vi "Build.vi"() -> ()   [LabVIEW 2014]
uses:
  <vilib>/AppBuilder/AB_API_Simple/Build Specification Version.ctl
  <vilib>/AppBuilder/AB_API_Simple/NI_App_Builder_API.lvlib
  <vilib>/AppBuilder/AB_API_Simple/Get Build Specification Version (path).vi
panel:
  out "Build Specification Version":T1
  out "Parent Directory (+ Relative)":path
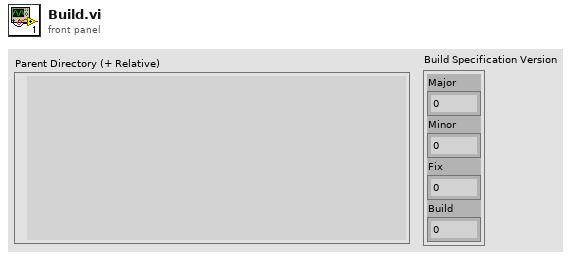
[diagram p1: front panel]
types:
  T1 = typedef "NI_App_Builder_API.lvlib/Build Specification Version.ctl" = cluster{"Major":u16, "Minor":u16, "Fix":u16, "Build":u16}
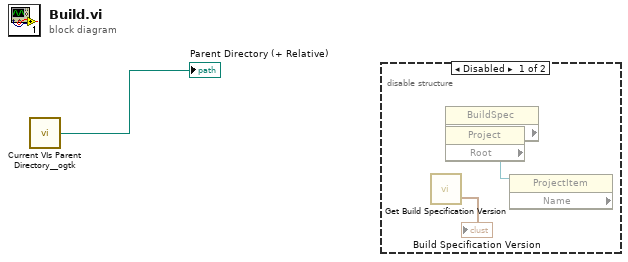
[diagram p0: block diagram]
diagram:
  n1 = call <userlib>:"Current VIs Parent Directory__ogtk.vi"() -> ("Parent Directory (+ Relative)"=→"Parent Directory (+ Relative)":path)  [unwired: 5 in]
  n2 = disable-structure shown="Disabled" {
    frame Disabled {
      n3 = call-poly <vilib>:"Get Build Specification Version.vi"() -> ("Build Specification Version"=→"Build Specification Version":T1)  [unwired: 10 in, 1 out]
      n4 = property class="BuildSpec" props=["Project"]() -> ()  [unwired: 2 in, 3 out]
      n5 = property class="Project"() -> ("Root"=w3:refnum<vi>)  [unwired: 2 in, 2 out]
      n6 = property class="ProjectItem" props=["Name"](reference=w3) -> ()  [unwired: 1 in, 3 out]
    }
    frame Enabled {
    }
  }
